vi "RemoveItemsBelongingToLibrary.vi"(9 "EvenSubLibraries":bool, 11 "LibraryDependency In":map{path, T1}(c390)) -> (3 "LibraryDependency Out":map{path, T1}(c390))   [LabVIEW 2020, in "DependencyChecker.lvlib"]
uses:
  DependencyChecker.lvlib
  LibraryDependentInfo.vi
  <vilib>/Utility/lvfile.llb/FT_FileTypes.ctl
  <vilib>/Utility/lvfile.llb/NI_FileType.lvlib
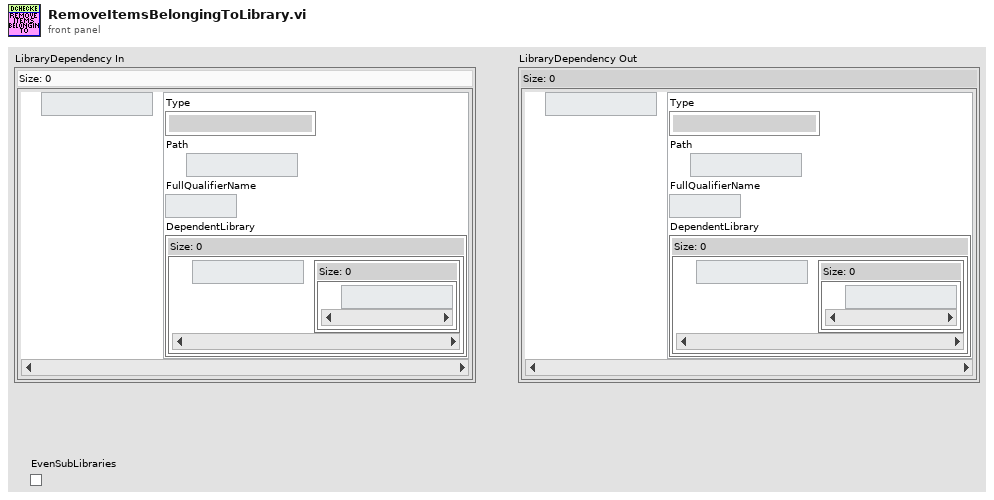
[diagram p1: front panel]
types:
  T1 = typedef "DependencyChecker.lvlib/LibraryDependentInfo.vi" = cluster{"Type":T2, "Path":path, "FullQualifierName":string, "DependentLibrary":map{path, set{path}}}
  T2 = typedef "NI_FileType.lvlib/FT_FileTypes.ctl" = enum32{"Invalid file/path", "Unknown type", "Instrument", "Control", "Polymorphic VI", "Project", "Library", "LVClass", "XControl", "XNode", "CIN", "Run-time menu", "Palette menu", "LLB", "Shortcut", "Directory", "Class Private Data Control", "Statechart", "MathScript .m file", "Ladder Diagram", "LVLibp"}
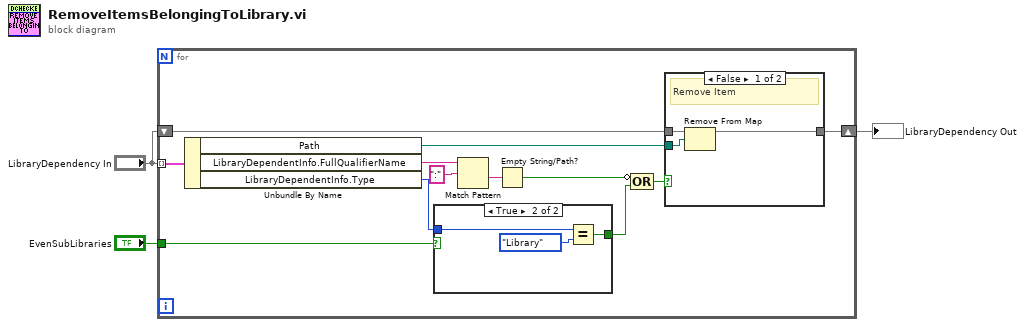
[diagram p0: block diagram]
diagram:
  n1 = for {
    tunnel: "LibraryDependency In" -> [w15] mode=indexing
    shift-right: [w12] -> w3
    shift-left: "LibraryDependency In" -> [w13]
    tunnel: "EvenSubLibraries" -> [w6]
    n2 = Unbundle By Name(w15) -> ("Path"=w11:path, "LibraryDependentInfo.FullQualifierName"=w10:string, "LibraryDependentInfo.Type"=w14:T2)
    n3 = case shown="True" w6 {
      tunnel: w14 -> [_ w18]
      tunnel: [_ w16] -> w5
      frame False {
      }
      frame True {
        n4 = Equal?(x=w18, y=FT_FileTypes."Library") -> (x = y?=w16:bool)
      }
    }
    n5 = Match Pattern(string=w10, regular expression=":") -> (after substring=w8:string)  [unwired: 1 in, 3 out]
    n6 = Empty String/Path?(string/path=w8) -> (empty?=w7:bool)
    n7 = Compound Arithmetic op=OR(invert w7, w5) -> (w4:bool)
    n8 = case shown="False" w4 {
      tunnel: w13 -> [w21 w22]
      tunnel: w11 -> [w20 _]
      tunnel: [w19 w22] -> w12
      frame False {
        # "Remove Item"
        n9 = Remove From Map(10:w20, 11:w21) -> (3:w19:map{path, T1})  [unwired: 2 out]
      }
      frame True {
        # "Keep this item"
      }
    }
  }
  "LibraryDependency Out" <- w3
